vi "lm Shut Down.vi"(8 "error in (no error)":errorcluster, 11 "hSerial":u32) -> (0 "error out":errorcluster, 3 "hSerial out":u32)   [LabVIEW 2017, in "LumencorDLLDbg64.lvlib"]
doc: "This function will close the Com port and release the resource for other applications use.\n\nextern \"C\" LUMENCORDLL2B_API void lmShutDown(HANDLE hSerial);"
uses:
  LumencorDLLDbg64.lvlib
  LumencorDLLDbg64.dll
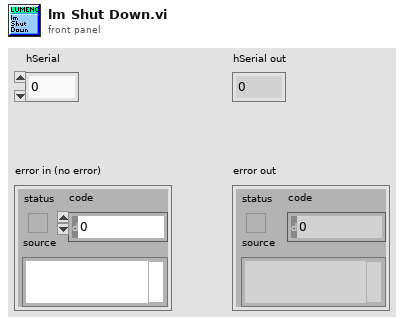
[diagram p1: front panel]
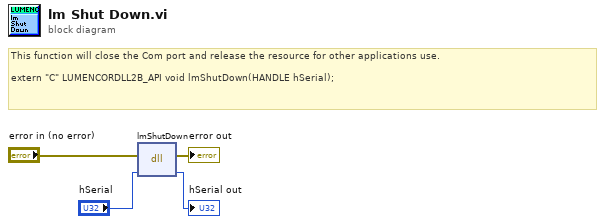
[diagram p0: block diagram]
diagram:
  # "This function will close the Com port and release the resource for other applications use.\n\nextern \"C\" LUMENCORDLL2B_API void lmShutDown(HANDLE hSerial);"
  n1 = dll-call lib="Q:/GIT -- Lumencor DLL4/LabVIEW Library (64bit)/LumencorDLLDbg64.*" fn="lmShutDown"(error in="error in (no error)", "hSerial"="hSerial") -> (error out=→"error out":errorcluster, "hSerial"=→"hSerial out":u32)  [unwired: 3 in, 1 out]
